vi "Sxx Measurements to Capacitance.vi"(7 "Sweep Frequency Start":dbl, 8 "error in (no error)":errorcluster, 11 "S11 Data":cdb[](array[numeric])) -> (0 "error out":errorcluster, 3 "Capacitance":dbl[](array[numeric]))   [LabVIEW 2013]
doc: "Converts the raw S11 data from niVNA fetch into capacitance measurement."
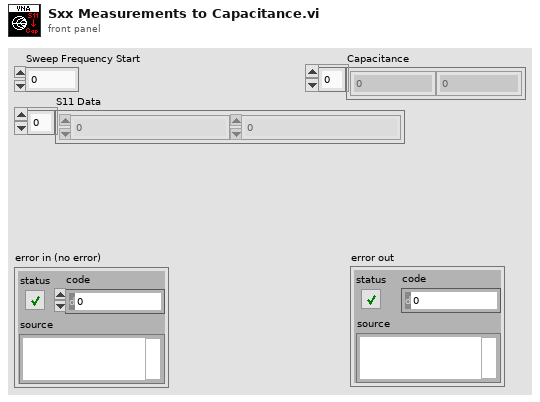
[diagram p1: front panel]
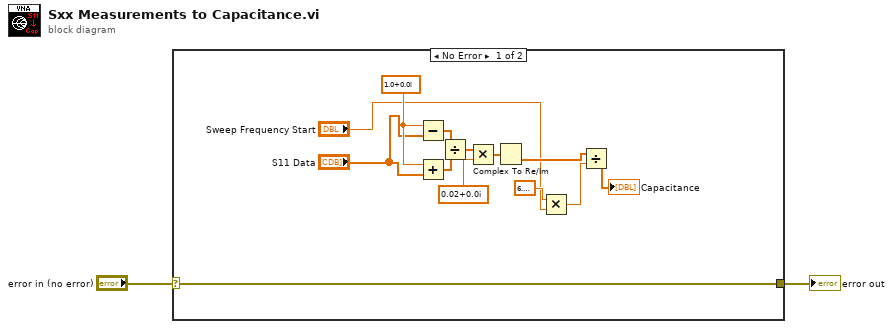
[diagram p0: block diagram]
diagram:
  n1 = case shown="No Error" "error in (no error)" {
    selector: "error in (no error)" -> [w15 w16]
    tunnel: [w15 w16] -> w2
    frame No Error {
      w14 = cdb 1.0+0.0i
      n2 = Subtract(x=w14, y="S11 Data") -> (x-y=w13:cdb[])
      n3 = Add(x=w14, y="S11 Data") -> (x+y=w12:cdb[])
      n4 = Divide(x=w13, y=w12) -> (x/y=w11:cdb[])
      n5 = Multiply(x=w11, y=cdb 0.02+0.0i) -> (x*y=w9:cdb[])
      n6 = Complex To Re/Im(x + iy=w9) -> (y=w7:dbl[])  [unwired: 1 out]
      n7 = Multiply(x=6.283185307179586, y="Sweep Frequency Start") -> (x*y=w6:dbl)
      n8 = Divide(x=w7, y=w6) -> (x/y=→"Capacitance":dbl[])
    }
    frame Error {
    }
  }
  "error out" <- w2
